vi "Automation_ERDS_Test.vi"(0 "GEA2 Reference In":refnum<k24>, 5 "GEA Inputs":T1 {"Destination" format="%.0x"; "Source" format="%.0x"}, 7 "Array_Test":T3(array[cluster]) {"ERD Number" format="%.0x"; "Time ms" min=100}, 11 "Error In":errorcluster) -> (4 "GEA2 Reference Out":refnum<k24>, 8 "Resultados":T2, 15 "Error Out":errorcluster)   [LabVIEW 2021]
uses:
  Type defs/Table_Result_Automation_Test.ctl
  Common/LabVIEW GEA2 Toolkit/GEA3/type defs/Source_Destination.ctl
  D:/Common/LabVIEW GEA2 Toolkit/source/GEA3 DLL Source/GeaCommunication.dll
  Common/LabVIEW GEA2 Toolkit/source/GEA3 DLL Source/GeaCommunication.dll
  Common/LabVIEW GEA2 Toolkit/GEA3/type defs/Data Type.ctl
  Common/LabVIEW GEA2 Toolkit/GEA3/type defs/ERD Write Data In.ctl
  Common/LabVIEW GEA2 Toolkit/GEA3/library/GEA2_Toolkit.lvlib
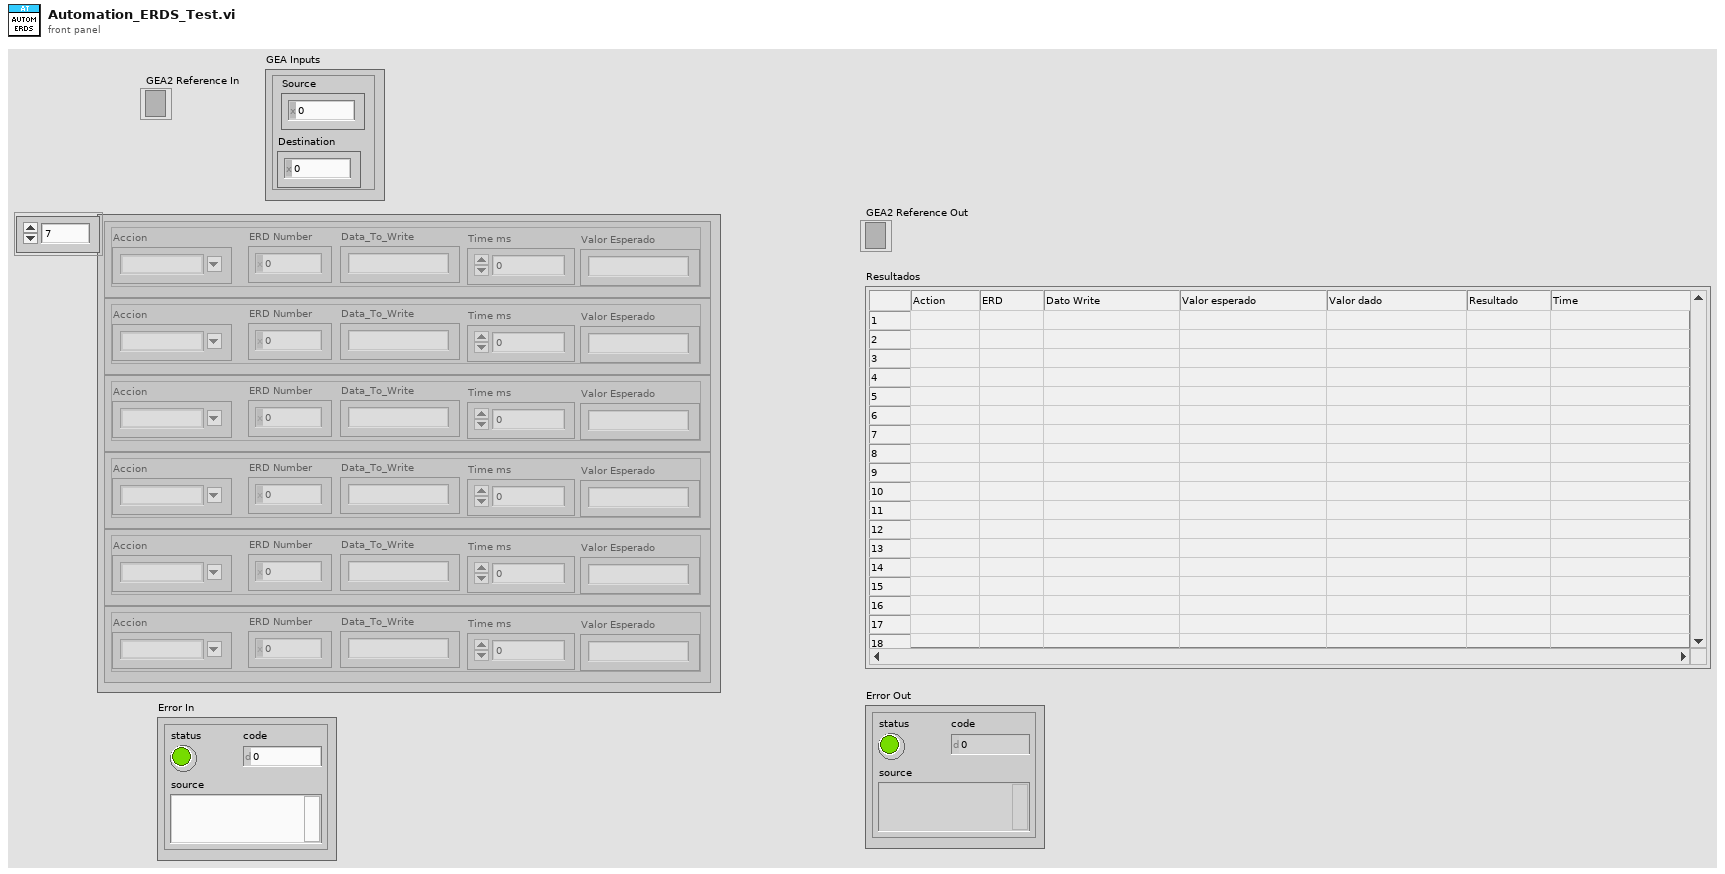
[diagram p1: front panel]
types:
  T1 = typedef "Source_Destination.ctl" = cluster{"Source":u8, "Destination":u8}
  T2 = typedef "Table_Result_Automation_Test.ctl" = string[][]
  T3 = cluster{"Accion":string, "Time ms":u32, "Valor Esperado":string, "ERD Number":u16, "Data_To_Write":string}[]
  T4 = typedef "Data Type.ctl" = enum16{"string", "boolean", "uint8_t", "uint16_t", "uint32_t", "uint64_t", "int8_t", "int16_t", "int32_t", "int64_t"}
  T5 = typedef "ERD Write Data In.ctl" = cluster{"ERD Number":u16, "Data Type":T4, "Data":string}
  T6 = cluster{"ERD Data Out[0]":cluster{"ERD Number":u16, "Data":string}, "ERD Data Out[1]":cluster{"ERD Number":u16, "Data":string}, "ERD Data Out[2]":cluster{"ERD Number":u16, "Data":string}, "ERD Data Out[3]":cluster{"ERD Number":u16, "Data":string}, "ERD Data Out[4]":cluster{"ERD Number":u16, "Data":string}, "ERD Data Out[5]":cluster{"ERD Number":u16, "Data":string}, "ERD Data Out[6]":cluster{"ERD Number":u16, "Data":string}, "ERD Data Out[7]":cluster{"ERD Number":u16, "Data":string}, "ERD Data Out[8]":cluster{"ERD Number":u16, "Data":string}}
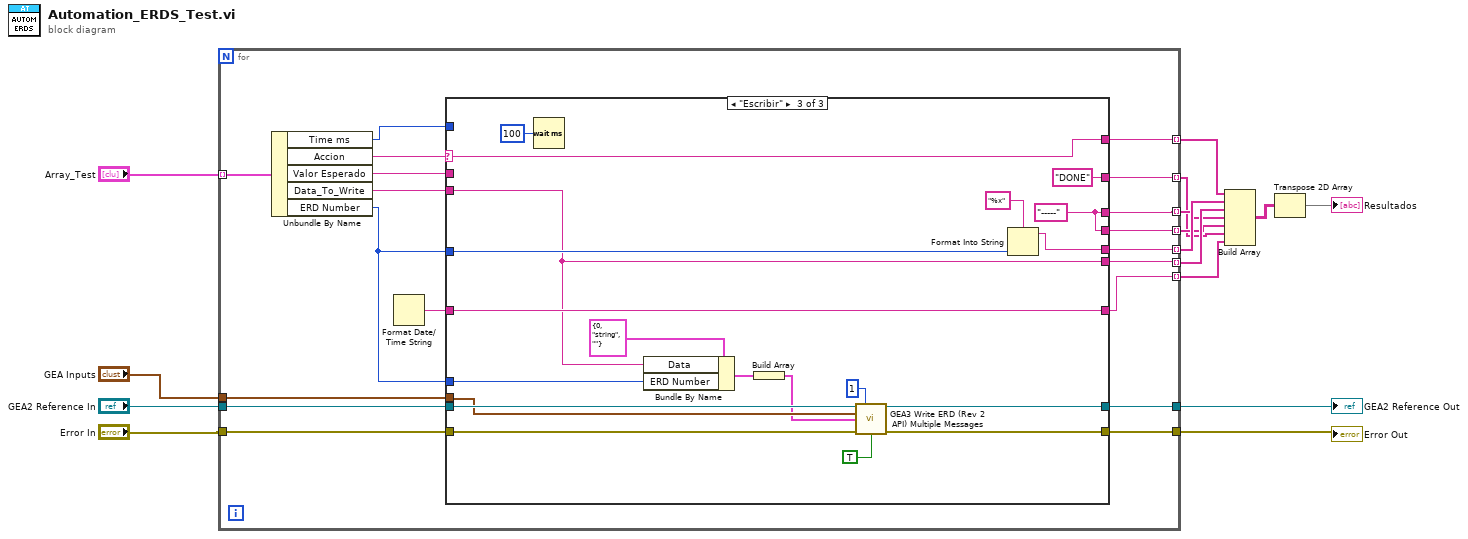
[diagram p0: block diagram]
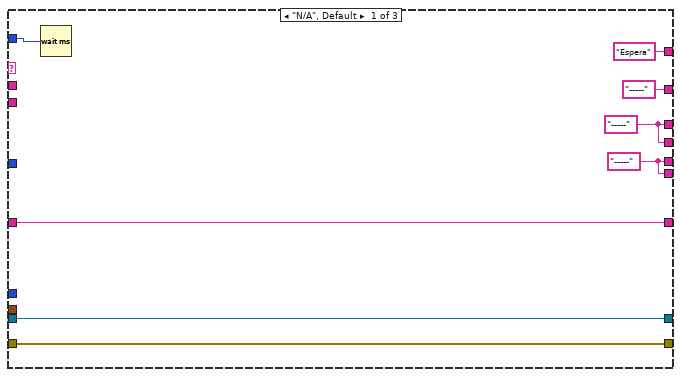
[diagram p2: hidden frame]
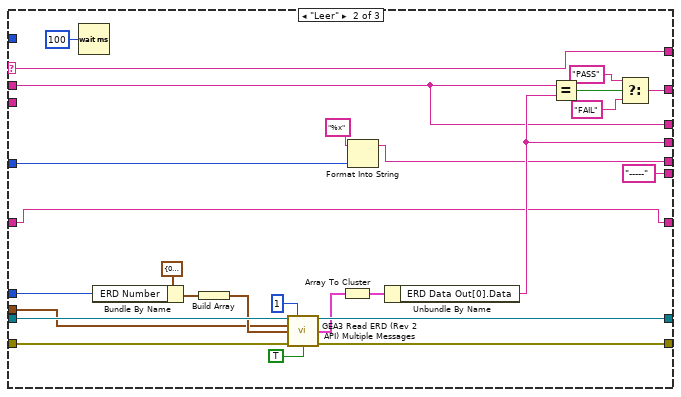
[diagram p3: hidden frame]
diagram:
  n1 = for {
    tunnel: "Array_Test" -> [w34] mode=indexing
    tunnel: "Error In" -> [w33]
    tunnel: "GEA2 Reference In" -> [w32]
    tunnel: [w31] -> w14
    tunnel: [w30] -> w13
    tunnel: "GEA Inputs" -> [w28]
    tunnel: [w25] -> w5 mode=indexing
    tunnel: [w24] -> w10 mode=indexing
    tunnel: [w23] -> w7 mode=indexing
    tunnel: [w22] -> w6 mode=indexing
    tunnel: [w20] -> w8 mode=indexing
    tunnel: [w19] -> w9 mode=indexing
    tunnel: [w17] -> w4 mode=indexing
    n2 = Unbundle By Name(w34) -> ("Time ms"=w16:u32, "Accion"=w29:string, "Valor Esperado"=w26:string, "Data_To_Write"=w27:string, "ERD Number"=w21:u16)
    n3 = Format Date/Time String() -> (date/time string=w18:string)  [unwired: 3 in]
    n4 = case shown="\"Escribir\"" w29 {
      selector: w29 -> [_ w51 w76]
      tunnel: w33 -> [w41 w68 w86]
      tunnel: w32 -> [w42 w67 w83]
      tunnel: [w42 w66 w84] -> w31
      tunnel: [w41 w65 w85] -> w30
      tunnel: w21 -> [_ w62 w80]
      tunnel: w28 -> [_ w60 w82]
      tunnel: w27 -> [_ _ w70]
      tunnel: w26 -> [_ w44 _]
      tunnel: ["-----" ("f") w52 "DONE" ("f")] -> w25
      tunnel: ["Espera" w51 w76] -> w24
      tunnel: [w39 w44 w75] -> w23
      tunnel: [w39 w50 w75] -> w22
      tunnel: w21 -> [_ w48 w74]
      tunnel: [w37 "-----" ("Data_To_Write") w70] -> w20
      tunnel: [w37 w47 w73] -> w19
      tunnel: [w36 w45 w71] -> w17
      tunnel: w18 -> [w36 w45 w71]
      tunnel: w16 -> [w35 _ _]
      frame "N/A", Default {
        w37 = "-----"
        w39 = "-----" ("Valor Esperado")
        n5 = Wait (ms)(milliseconds to wait=w35) -> ()  [unwired: 1 out]
      }
      frame "Leer" {
        n6 = Wait (ms)(milliseconds to wait=u32 100) -> ()  [unwired: 1 out]
        n7 = Bundle By Name(cluster=cluster{"ERD Number":u16, "Data Type":T4} {"ERD Number"=0, "Data Type"=enum."string"} ("ERD Read Data In"), "ERD Number"=w62) -> (w64:cluster{"ERD Number":u16, "Data Type":T4})
        n8 = Build Array(w64) -> (w61:cluster{"ERD Number":u16, "Data Type":T4}[])
        n9 = call "GEA3 Read ERD (Rev 2 API) Multiple Messages.vi"("GEA2 Reference In"=w67, "Retry Count"=1, "GEA Inputs"=w60, "Read ERD List"=w61, "Error In"=w68, "Verify ERD Response?"=TRUE) -> ("GEA2 Reference Out"=w66:refnum<k24>, "ERD Data Out"=w57:cluster{"ERD Number":u16, "Data":string}[], "Error Out"=w65:errorcluster)  [unwired: 6 in, 1 out]
        n10 = Array To Cluster(array=w57) -> (cluster=w56:T6)
        n11 = Format Into String(format string="%x", w48) -> (resulting string=w47:string)  [unwired: 2 in, 1 out]
        n12 = Unbundle By Name(w56) -> ("ERD Data Out[0].Data"=w50:string)
        n13 = Equal?(x=w44, y=w50) -> (x = y?=w55:bool)
        n14 = Select(t="PASS" ("String"), s=w55, f="FAIL") -> (s? t:f=w52:string)
      }
      frame "Escribir" {
        w75 = "-----" ("Valor Esperado")
        n15 = Wait (ms)(milliseconds to wait=u32 100) -> ()  [unwired: 1 out]
        n16 = Bundle By Name(cluster=T5 {"ERD Number"=0, "Data Type"=enum."string", "Data"=""} ("ERD Write Data In"), "Data"=w70, "ERD Number"=w80) -> (w79:T5)
        n17 = Build Array(w79) -> (w78:T5[])
        n18 = call "GEA3 Write ERD (Rev 2 API) Multiple Messages.vi"("GEA2 Reference In"=w83, "# of Tries"=1 ("Retry Count"), "GEA Inputs"=w82, "Write ERD List"=w78, "Error In"=w86, "Verify ERD Response?"=TRUE) -> ("GEA2 Reference Out"=w84:refnum<k24>, "Error Out"=w85:errorcluster)  [unwired: 7 in, 1 out]
        n19 = Format Into String(format string="%x", w74) -> (resulting string=w73:string)  [unwired: 2 in, 1 out]
      }
    }
  }
  "GEA2 Reference Out" <- w14
  "Error Out" <- w13
  n20 = Build Array(w10, w9, w8, w7, w6, w5, w4) -> (w12:string[][])
  n21 = Transpose 2D Array(2D array=w12) -> (transposed array=→"Resultados":string[][])
